vi "worksheet write rich string.vi"(6 "format":u32, 7 "rich_string":u32, 8 "error in (no error)":errorcluster, 9 "col":u16, 10 "row":u32, 11 "worksheet":u32) -> (0 "error out":errorcluster, 3 "function return":u32(ring))   [LabVIEW 2015, in "xlsxwriter.lvlib"]
doc: "lxw_error worksheet_write_rich_string(lxw_worksheet worksheet, lxw_row_t row, lxw_col_t col, unsigned long rich_string, lxw_format format);"
uses:
  xlsxwriter.lvlib
  xlsxwriter.dll
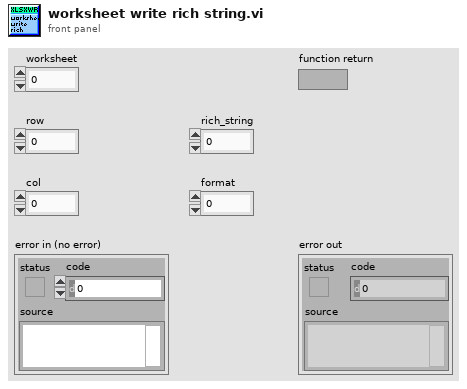
[diagram p1: front panel]
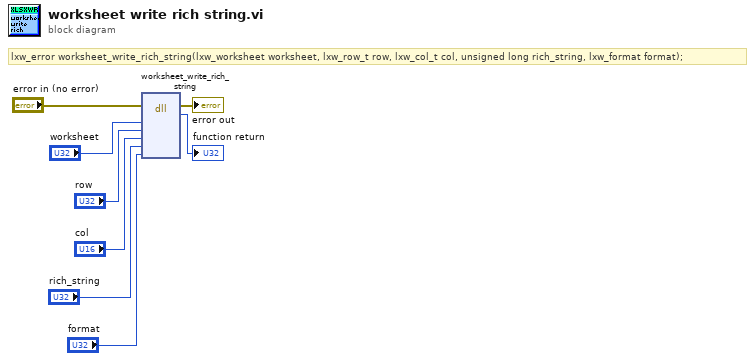
[diagram p0: block diagram]
diagram:
  # "lxw_error worksheet_write_rich_string(lxw_worksheet worksheet, lxw_row_t row, lxw_col_t col, unsigned long rich_string, lxw_format format);"
  n1 = dll-call lib="C:/Users/WDAGUtilityAccount/Desktop/lv_vis_added_cell/xlsxwriter.*" fn="worksheet_write_rich_string"(error in="error in (no error)", "worksheet"="worksheet", "row"="row", "col"="col", "rich_string"="rich_string", "format"="format") -> (error out=→"error out":errorcluster, →"function return":u32)  [unwired: 7 in, 1 out]
